vi "FarFiledCorrectArea.vi"(0 "X中心坐标序列":dbl[](array[numeric]), 1 "X面积序列":dbl[](array[numeric]), 2 "Y中心坐标序列":dbl[](array[numeric]), 3 "Y面积序列":dbl[](array[numeric]), 4 "位置坐标":dbl[](array[numeric])) -> (6 "X校正面积输出":dbl[](array[numeric]), 7 "Y校正面积输出":dbl[](array[numeric]))   [LabVIEW 2018]
uses:
  <vilib>/Analysis/NI_AALPro.lvlib
panel:
  out "arctan(x)":dbl
  out "slope":dbl caption="斜率"
  out "XY图":cluster{"位置坐标":dbl[], "Best Linear Fit":dbl[]}[](graph)
  # "修正因为角度偏移造成的面积偏移，估计出夹角后面积反投影至实际大小"
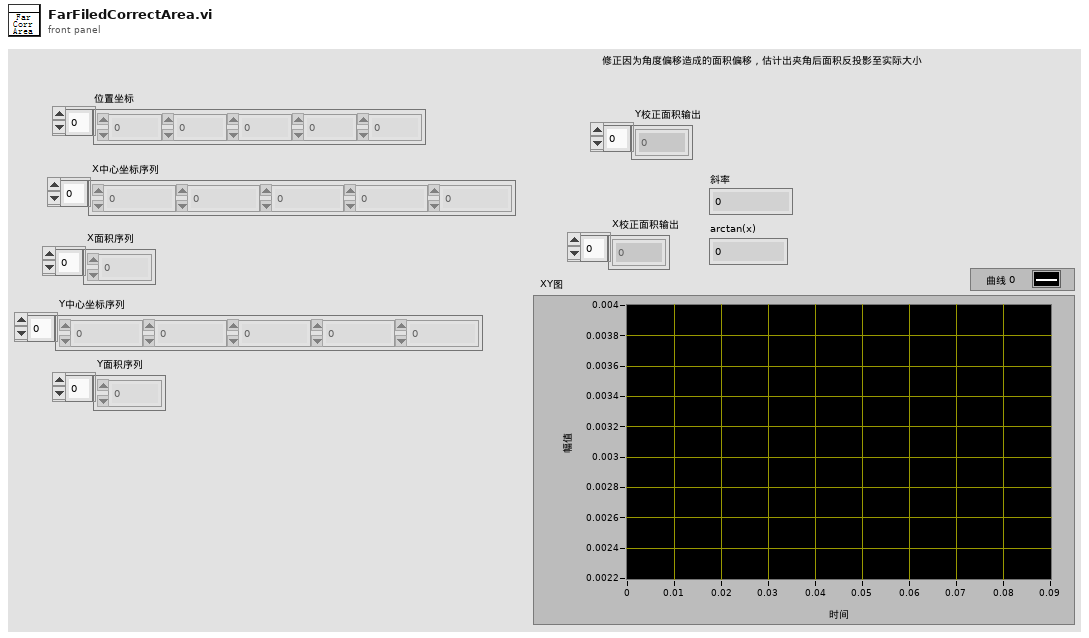
[diagram p1: front panel]
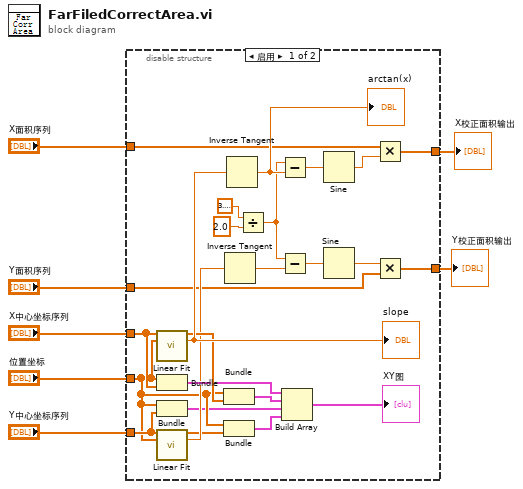
[diagram p0: block diagram]
diagram:
  n1 = disable-structure shown="启用" {
    disable-tunnel: "位置坐标" -> [w11 _]
    disable-tunnel: "X中心坐标序列" -> [w24 _]
    disable-tunnel: "X面积序列" -> [w27 w34]
    disable-tunnel: [w25 w34] -> w4
    disable-tunnel: "Y中心坐标序列" -> [w12 _]
    disable-tunnel: "Y面积序列" -> [w14 w33]
    disable-tunnel: [w13 w33] -> w1
    frame Enabled {
      n2 = call <vilib>:"Linear Fit.vi"("Y"=w24, "X"=w11) -> ("Best Linear Fit"=w23:dbl[], "slope"=w32:dbl)  [unwired: 9 in, 3 out]
      "slope" <- w32
      n3 = Bundle("位置坐标"=w11, "X中心坐标序列"=w24) -> (w22:cluster{"位置坐标":dbl[], " X中心坐标序列":dbl[]})  [unwired: 1 in]
      n4 = Bundle("位置坐标"=w11, "Y中心坐标序列"=w12) -> (w9:cluster{"位置坐标":dbl[], " Y中心坐标序列":dbl[]})  [unwired: 1 in]
      n5 = call <vilib>:"Linear Fit.vi"("Y"=w12, "X"=w11) -> ("Best Linear Fit"=w10:dbl[], "slope"=w19:dbl)  [unwired: 9 in, 3 out]
      n6 = Bundle("位置坐标"=w11, "Best Linear Fit"=w23) -> (w21:cluster{"位置坐标":dbl[], "Best Linear Fit":dbl[]})  [unwired: 1 in]
      n7 = Bundle("位置坐标"=w11, "Best Linear Fit"=w10) -> (w8:cluster{"位置坐标":dbl[], "Best Linear Fit":dbl[]})  [unwired: 1 in]
      n8 = Inverse Tangent(1:w19) -> (0:w17:dbl)
      n9 = Inverse Tangent(1:w32) -> (0:w29:dbl)
      "arctan(x)" <- w29
      n10 = Divide(x=3.141592653589793, y=2.0) -> (x/y=w18:dbl)
      n11 = Subtract(x=w18, y=w29) -> (x-y=w28:dbl)
      n12 = Subtract(x=w18, y=w17) -> (x-y=w16:dbl)
      n13 = Build Array(w22, w21, w9, w8) -> (→"XY图":cluster{"位置坐标":dbl[], "Best Linear Fit":dbl[]}[])
      n14 = Sine(x=w28) -> (sin(x)=w26:dbl)
      n15 = Sine(x=w16) -> (sin(x)=w15:dbl)
      n16 = Multiply(x=w27, y=w26) -> (x*y=w25:dbl[])
      n17 = Multiply(x=w15, y=w14) -> (x*y=w13:dbl[])
    }
    frame Disabled {
    }
  }
  "X校正面积输出" <- w4
  "Y校正面积输出" <- w1
